vi "currentSet_FGV.vi"(7 "Enum":enum16{"set", "read"}(ring), 11 "curent set":u16) -> (3 "curent set out":u16)   [LabVIEW 2013]
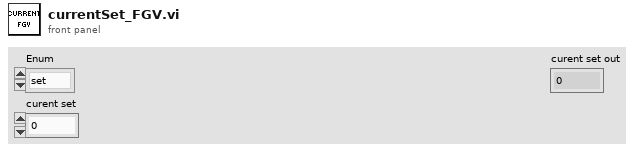
[diagram p1: front panel]
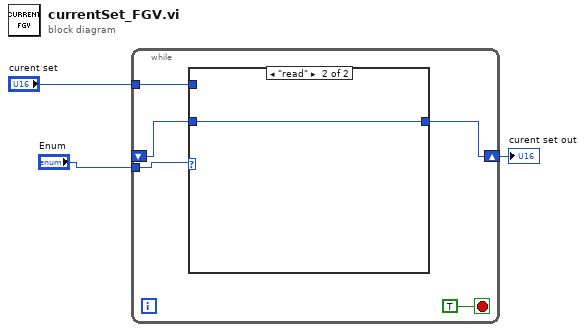
[diagram p0: block diagram]
diagram:
  n1 = while {
    shift-right: [w6] -> w1
    shift-left: _ -> [w4]
    tunnel: "Enum" -> [w7]
    tunnel: "curent set" -> [w5]
    stop <- TRUE stop-if-true
    n2 = case shown="\"read\"" w7 {
      tunnel: [w9 w10] -> w6
      tunnel: w5 -> [w9 _]
      tunnel: w4 -> [_ w10]
      frame "set" {
      }
      frame "read" {
      }
    }
  }
  "curent set out" <- w1
